vi "Teleop.vi"(10 "Match Info":T1={"Autonomous Elapsed Seconds"=0.0, "TeleOp Elapsed Seconds"=0.0, "Disabled Elapsed Seconds"=0.0, "Visited Autonomous"=FALSE, "Visited TeleOp"=FALSE, "Visited Disabled"=FALSE, "Autonomous Settings"={"Autonomous Style"=enum."Independent", "VI Refnum"=refnum}}, 11 "Call Context":T2) -> ()   [LabVIEW 2019]
doc: "This VI is called for each enabled TeleOp packet received from the DS. It is typically used to read from joysticks and other inputs and update I/O or setpoints for timed control loops. It should complete and return within 20 milliseconds or risk missing DS packets."
uses:
  <vilib>/Rock Robotics/WPI/DriverStation/WPI_DriverStationDerivedRobotMode.ctl
  <vilib>/Rock Robotics/WPI/DriverStation/WPI_DriverStationMatch Info.ctl
  Framework/Robot Global Data.vi
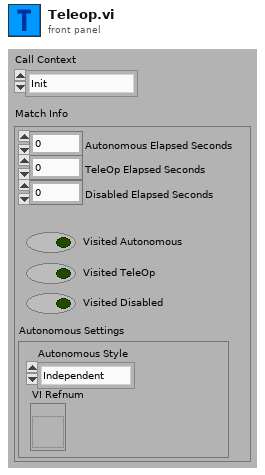
[diagram p1: front panel]
types:
  T1 = typedef "WPI_DriverStationMatch Info.ctl" = cluster{"Autonomous Elapsed Seconds":dbl, "TeleOp Elapsed Seconds":dbl, "Disabled Elapsed Seconds":dbl, "Visited Autonomous":bool, "Visited TeleOp":bool, "Visited Disabled":bool, "Autonomous Settings":cluster{"Autonomous Style":enum16{"Iterative", "Independent"}, "VI Refnum":refnum<vi>}}
  T2 = typedef "WPI_DriverStationDerivedRobotMode.ctl" = enum16{"Init", "Execute", "Stop"}
  T3 = typedef "Command Status Info.ctl" = cluster{"Name":string, "Status":T4, "notifier out":T5}
  T4 = typedef "Completion Status.ctl" = enum16{"Successful", "Aborted", "Incomplete"}
  T5 = typedef "Completion Notifier.ctl" = refnum<notifier>
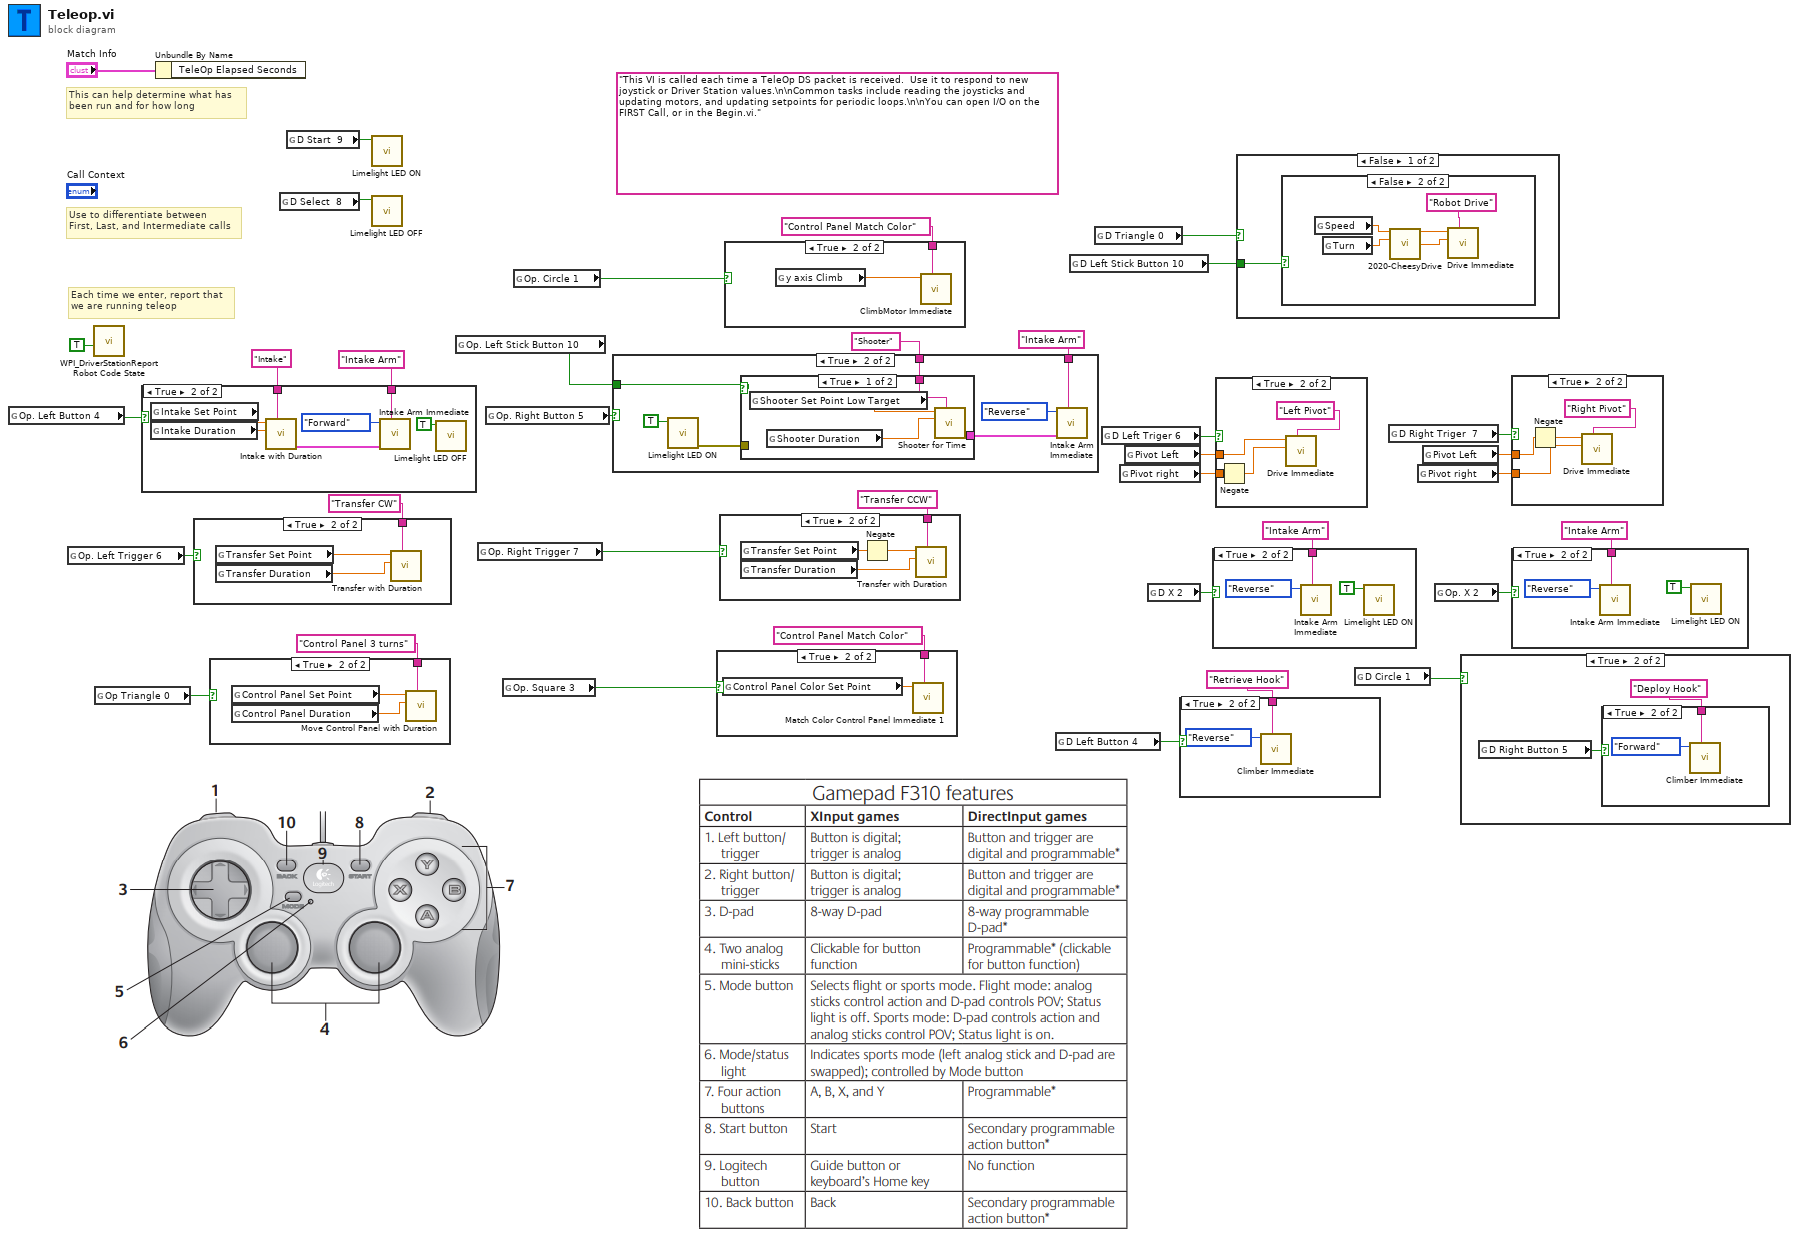
[diagram p0: block diagram]
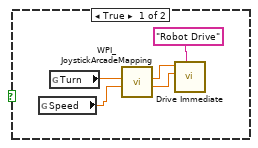
[diagram p7: hidden frame]
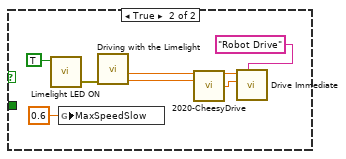
[diagram p8: hidden frame]
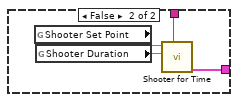
[diagram p17: hidden frame]
diagram:
  (unwired) "This VI is called each time a TeleOp DS packet is received.  Use it to respond to new joystick or Driver Station values.\n\nCommon tasks include reading the joysticks and updating motors, and updating setpoints for periodic loops.\n\nYou can open I/O on the FIRST Call, or in the Begin.vi."
  # "Each time we enter, report that\nwe are running teleop"
  # "Use to differentiate between\nFirst, Last, and Intermediate calls"
  # "This can help determine what has\nbeen run and for how long"
  n1 = global read "Robot Global Data.vi" "Op. Left Button 4"() -> (w34:bool)
  n2 = global read "Robot Global Data.vi" "Op. Left Trigger 6"() -> (w28:bool)
  n3 = call <vilib>:"WPI_DriverStationReport Robot Code State.vi"("TeleOp"=TRUE ("Autonomous")) -> ()  [unwired: 10 in, 1 out]
  n4 = global read "Robot Global Data.vi" "Op Triangle 0"() -> (w21:bool)
  n5 = case shown="True" w34 {
    tunnel: "Intake" ("refnum name") -> [_ w43]
    tunnel: "Intake Arm" ("refnum name") -> [_ w39]
    frame False {
    }
    frame True {
      n6 = global read "Robot Global Data.vi" "Intake Set Point"() -> (w42:dbl)
      n7 = global read "Robot Global Data.vi" "Intake Duration"() -> (w41:dbl)
      n8 = call "Intake with Duration.vi"("Description"=w43, "Duration (s)"=w41, "Setpoint"=w42) -> ("Command Info Out"=w38:T3)  [unwired: 8 in]
      n9 = call "Intake Arm Immediate.vi"("Description"=w39, "Command Info In"=w38, "Relay Value"=enum16{"Off", "On", "Forward", "Reverse"}."Forward") -> ()  [unwired: 8 in, 1 out]
      n10 = call "Limelight LED OFF.vi"("D Select  8"=TRUE) -> ()  [unwired: 11 in]
    }
  }
  n11 = Unbundle By Name("Match Info") -> ()  [unwired: 1 out]
  n12 = case shown="True" w28 {
    tunnel: "Transfer CW" ("refnum name") -> [_ w46]
    frame False {
    }
    frame True {
      n13 = global read "Robot Global Data.vi" "Transfer Set Point"() -> (w45:dbl)
      n14 = global read "Robot Global Data.vi" "Transfer Duration"() -> (w44:dbl)
      n15 = call "Transfer with Duration.vi"("Description"=w46, "Duration (s)"=w44, "Setpoint"=w45) -> ()  [unwired: 8 in, 1 out]
    }
  }
  n16 = case shown="True" w21 {
    tunnel: "Control Panel 3 turns" ("refnum name") -> [_ w49]
    frame False {
    }
    frame True {
      n17 = global read "Robot Global Data.vi" "Control Panel Set Point"() -> (w48:dbl)
      n18 = global read "Robot Global Data.vi" "Control Panel Duration"() -> (w47:dbl)
      n19 = call "Move Control Panel with Duration.vi"("Description"=w49, "Duration (s)"=w47, "Setpoint"=w48) -> ()  [unwired: 8 in, 1 out]
    }
  }
  n20 = global read "Robot Global Data.vi" "D Select  8"() -> (w2:bool)
  n21 = global read "Robot Global Data.vi" "D Start  9"() -> (w3:bool)
  n22 = call "Limelight LED ON.vi"("D Start  9"=w3) -> ()  [unwired: 10 in, 1 out]
  n23 = call "Limelight LED OFF.vi"("D Select  8"=w2) -> ()  [unwired: 11 in]
  n24 = global read "Robot Global Data.vi" "Op. Left Stick Button 10"() -> (w4:bool)
  n25 = global read "Robot Global Data.vi" "Op. Right Trigger 7"() -> (w29:bool)
  n26 = global read "Robot Global Data.vi" "Op. Right Button 5"() -> (w30:bool)
  n27 = global read "Robot Global Data.vi" "Op. Square 3"() -> (w18:bool)
  n28 = global read "Robot Global Data.vi" "Op. Circle 1"() -> (w6:bool)
  n29 = case shown="True" w30 {
    tunnel: "Shooter" ("refnum name") -> [_ w56]
    tunnel: "Intake Arm" ("refnum name") -> [_ w54]
    tunnel: w4 -> [_ w52]
    frame False {
    }
    frame True {
      n30 = call "Limelight LED ON.vi"("D Start  9"=TRUE) -> ("error out"=w50:errorcluster)  [unwired: 10 in]
      n31 = case shown="True" w52 {
        tunnel: w56 -> [w60 w64]
        tunnel: [w57 w61] -> w53
        tunnel: w50 -> [_ _]
        frame True {
          n32 = global read "Robot Global Data.vi" "Shooter Set Point Low Target"() -> (w59:dbl)
          n33 = global read "Robot Global Data.vi" "Shooter Duration"() -> (w58:dbl)
          n34 = call "Shooter for Time.vi"("Description"=w60, "Duration (s)"=w58, "Setpoint"=w59) -> ("Command Info Out"=w57:T3)  [unwired: 8 in]
        }
        frame False {
          n35 = global read "Robot Global Data.vi" "Shooter Set Point"() -> (w63:dbl)
          n36 = global read "Robot Global Data.vi" "Shooter Duration"() -> (w62:dbl)
          n37 = call "Shooter for Time.vi"("Description"=w64, "Duration (s)"=w62, "Setpoint"=w63) -> ("Command Info Out"=w61:T3)  [unwired: 8 in]
        }
      }
      n38 = call "Intake Arm Immediate.vi"("Description"=w54, "Command Info In"=w53, "Relay Value"=enum16{"Off", "On", "Forward", "Reverse"}."Reverse") -> ()  [unwired: 8 in, 1 out]
    }
  }
  n39 = case shown="True" w18 {
    tunnel: "Control Panel Match Color" ("refnum name") -> [_ w66]
    frame False {
    }
    frame True {
      n40 = global read "Robot Global Data.vi" "Control Panel Color Set Point"() -> (w65:dbl)
      n41 = call "Match Color Control Panel Immediate 1.vi"("Description"=w66, "Setpoint"=w65) -> ()  [unwired: 9 in, 1 out]
    }
  }
  n42 = case shown="True" w29 {
    tunnel: "Transfer CCW" ("refnum name") -> [_ w70]
    frame False {
    }
    frame True {
      n43 = global read "Robot Global Data.vi" "Transfer Set Point"() -> (w68:dbl)
      n44 = global read "Robot Global Data.vi" "Transfer Duration"() -> (w67:dbl)
      n45 = Negate(x=w68) -> (-x=w69:dbl)
      n46 = call "Transfer with Duration.vi"("Description"=w70, "Duration (s)"=w67, "Setpoint"=w69) -> ()  [unwired: 8 in, 1 out]
    }
  }
  n47 = case shown="True" w6 {
    tunnel: "Control Panel Match Color" ("refnum name") -> [_ w72]
    frame False {
    }
    frame True {
      n48 = global read "Robot Global Data.vi" "y axis Climb"() -> (w71:dbl)
      n49 = call "ClimbMotor Immediate.vi"("Description"=w72, "Setpoint"=w71) -> ()  [unwired: 9 in, 1 out]
    }
  }
  n50 = global read "Robot Global Data.vi" "D Left Button 4"() -> (w11:bool)
  n51 = global read "Robot Global Data.vi" "D Left Stick Button 10"() -> (w1:bool)
  n52 = global read "Robot Global Data.vi" "D Triangle 0"() -> (w12:bool)
  n53 = global read "Robot Global Data.vi" "D Left Triger 6"() -> (w26:bool)
  n54 = global read "Robot Global Data.vi" "Pivot right"() -> (w15:dbl)
  n55 = global read "Robot Global Data.vi" "Pivot Left"() -> (w16:dbl)
  n56 = global read "Robot Global Data.vi" "D X 2"() -> (w19:bool)
  n57 = case shown="True" w11 {
    tunnel: "Retrieve Hook" ("refnum name") -> [_ w73]
    frame False {
    }
    frame True {
      n58 = call "Climber Immediate.vi"("Description"=w73, "Value"=enum16{"Off", "On", "Forward", "Reverse"}."Reverse" ("Relay Value")) -> ()  [unwired: 9 in, 1 out]
    }
  }
  n59 = case shown="True" w19 {
    tunnel: "Intake Arm" ("refnum name") -> [_ w76]
    frame False {
    }
    frame True {
      n60 = call "Intake Arm Immediate.vi"("Description"=w76, "Relay Value"=enum16{"Off", "On", "Forward", "Reverse"}."Reverse") -> ()  [unwired: 9 in, 1 out]
      n61 = call "Limelight LED ON.vi"("D Start  9"=TRUE) -> ()  [unwired: 10 in, 1 out]
    }
  }
  n62 = case shown="True" w26 {
    tunnel: w16 -> [_ w80]
    tunnel: w15 -> [_ w79]
    frame False {
    }
    frame True {
      n63 = Negate(x=w79) -> (-x=w78:dbl)
      n64 = call "Drive Immediate.vi"("Description"="Left Pivot", "Right Setpoint"=w78, "Left Setpoint"=w80) -> ()  [unwired: 8 in, 1 out]
    }
  }
  n65 = case shown="False" w12 {
    tunnel: w1 -> [w82 _]
    frame False {
      n66 = case shown="False" w82 {
        frame True {
          n67 = global read "Robot Global Data.vi" "Speed"() -> (w85:dbl)
          n68 = global read "Robot Global Data.vi" "Turn"() -> (w86:dbl)
          n69 = call <vilib>:"WPI_JoystickArcadeMapping.vi"("Y axis value"=w85, "X axis value"=w86) -> ("Right Motor Value"=w83:dbl, "Left Motor Value"=w84:dbl)  [unwired: 8 in]
          n70 = call "Drive Immediate.vi"("Description"="Robot Drive", "Right Setpoint"=w83, "Left Setpoint"=w84) -> ()  [unwired: 8 in, 1 out]
        }
        frame False {
          n71 = global read "Robot Global Data.vi" "Speed"() -> (w89:dbl)
          n72 = global read "Robot Global Data.vi" "Turn"() -> (w90:dbl)
          n73 = call "2020-CheesyDrive.vi"("Throttle"=w89, "Wheel"=w90) -> ("Left PWM"=w91:dbl, "Right PWM"=w92:dbl)  [unwired: 12 in]
          n74 = call "Drive Immediate.vi"("Description"="Robot Drive", "Right Setpoint"=w92, "Left Setpoint"=w91) -> ()  [unwired: 8 in, 1 out]
        }
      }
    }
    frame True {
      n75 = call "Limelight LED ON.vi"("D Start  9"=TRUE) -> ("error out"=w95:errorcluster)  [unwired: 10 in]
      n76 = global write "Robot Global Data.vi" "MaxSpeedSlow"(0.6 ("MaxSpeedSlow")) -> ()
      n77 = call "Driving with the Limelight.vi"("error in (no error)"=w95) -> ("TurnCommand"=w96:dbl, "SpeedCommand"=w97:dbl)  [unwired: 8 in, 1 out]
      n78 = call "2020-CheesyDrive.vi"("Throttle"=w97, "Wheel"=w96) -> ("Left PWM"=w99:dbl, "Right PWM"=w100:dbl)  [unwired: 12 in]
      n79 = call "Drive Immediate.vi"("Description"="Robot Drive", "Right Setpoint"=w100, "Left Setpoint"=w99) -> ()  [unwired: 8 in, 1 out]
    }
  }
  n80 = global read "Robot Global Data.vi" "D Circle 1"() -> (w5:bool)
  n81 = global read "Robot Global Data.vi" "D Right Triger  7"() -> (w25:bool)
  n82 = global read "Robot Global Data.vi" "Pivot right"() -> (w13:dbl)
  n83 = global read "Robot Global Data.vi" "Pivot Left"() -> (w14:dbl)
  n84 = global read "Robot Global Data.vi" "Op. X 2"() -> (w9:bool)
  n85 = case shown="True" w5 {
    frame False {
    }
    frame True {
      n86 = global read "Robot Global Data.vi" "D Right Button 5"() -> (w101:bool)
      n87 = case shown="True" w101 {
        tunnel: "Deploy Hook" ("refnum name") -> [_ w103]
        frame False {
        }
        frame True {
          n88 = call "Climber Immediate.vi"("Description"=w103, "Value"=enum16{"Off", "On", "Forward", "Reverse"}."Forward" ("Relay Value")) -> ()  [unwired: 9 in, 1 out]
        }
      }
    }
  }
  n89 = case shown="True" w25 {
    tunnel: w14 -> [_ w107]
    tunnel: w13 -> [_ w106]
    frame False {
    }
    frame True {
      n90 = Negate(x=w107) -> (-x=w105:dbl)
      n91 = call "Drive Immediate.vi"("Description"="Right Pivot", "Right Setpoint"=w106, "Left Setpoint"=w105) -> ()  [unwired: 8 in, 1 out]
    }
  }
  n92 = case shown="True" w9 {
    tunnel: "Intake Arm" ("refnum name") -> [_ w110]
    frame False {
    }
    frame True {
      n93 = call "Intake Arm Immediate.vi"("Description"=w110, "Relay Value"=enum16{"Off", "On", "Forward", "Reverse"}."Reverse") -> ()  [unwired: 9 in, 1 out]
      n94 = call "Limelight LED ON.vi"("D Start  9"=TRUE) -> ()  [unwired: 10 in, 1 out]
    }
  }
